vi "R4DOControl.vi"(8 "error constant":errorcluster, 11 "LabVIEW Web Service":refnum<class "Web Service.lvclass">) -> ()   [LabVIEW 2016]
uses:
  <vilib>/wsapi/Web Service.lvclass
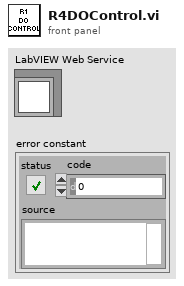
[diagram p1: front panel]
types:
  T1 = cluster{"Media Pump":bool, "Water Pump":bool, "Gas Pump":bool, "Effluent Pump":bool, "Release Pump":bool}
  T2 = cluster{"Set Point, mg/L":dbl, "Tolerance, mg/L":dbl, "N2 Valve Gain":dbl, "Air Valve Gain":dbl}
  T3 = cluster{"Signal, mA":dbl, "Value, UNITS HERE":dbl}
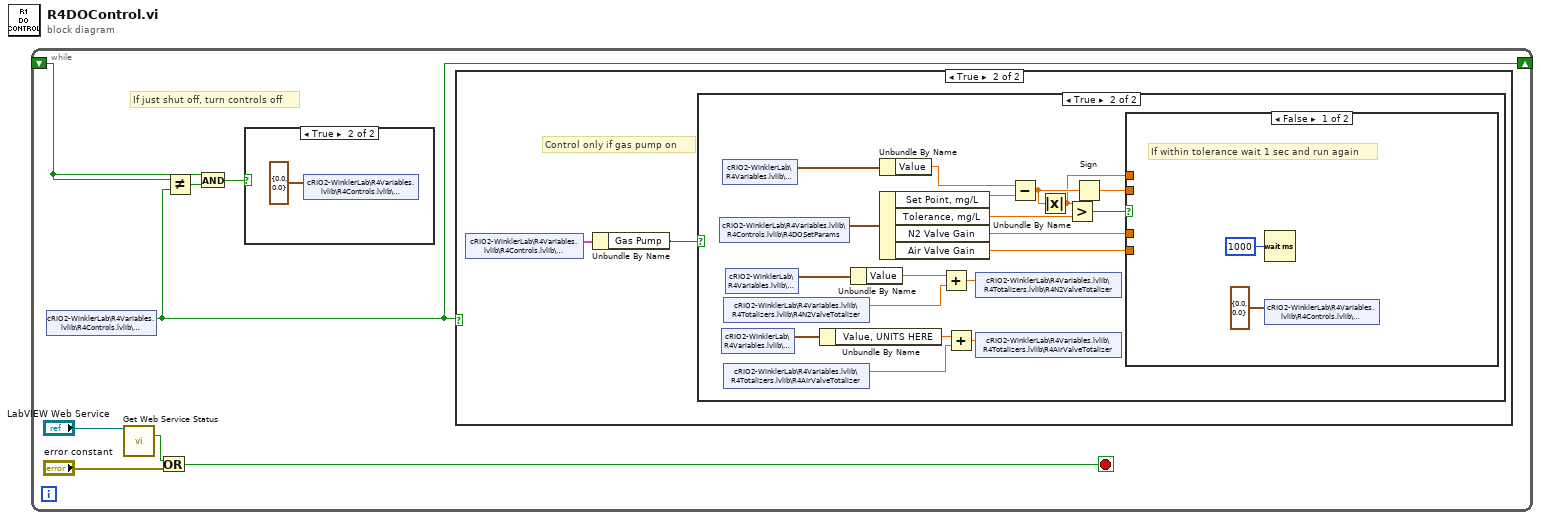
[diagram p0: block diagram]
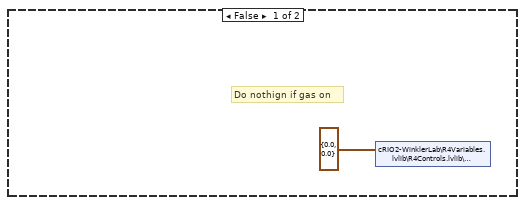
[diagram p4: hidden frame]
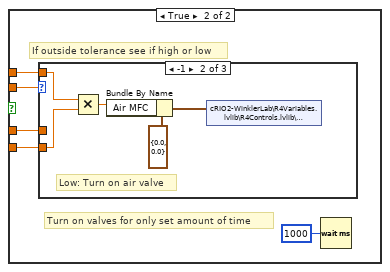
[diagram p5: hidden frame]
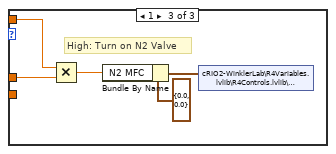
[diagram p7: hidden frame]
diagram:
  n1 = while {
    shift-right: [w1] -> _
    shift-left: _ -> [w2]
    stop <- w5 stop-if-true
    # "If just shut off, turn controls off"
    n2 = shared-variable "cRIO2-WinklerLab\\R4Variables.lvlib\\R4Controls.lvlib\\R4DOSwitch"() -> (w1:bool)  [unwired: 1 in, 1 out]
    n3 = call <vilib>:"Get Web Service Status.vi"("LabVIEW Web Service"="LabVIEW Web Service") -> ("service stopping?"=w8:bool)  [unwired: 12 in, 2 out]
    n4 = Or(x=w8, y="error constant") -> (x .or. y?=w5:bool)
    n5 = Not Equal?(x=w2, y=w1) -> (x != y?=w3:bool)
    n6 = And(x=w2, y=w3) -> (x .and. y?=w4:bool)
    n7 = case shown="True" w4 {
      frame False {
      }
      frame True {
        n8 = shared-variable "cRIO2-WinklerLab\\R4Variables.lvlib\\R4Controls.lvlib\\R4DOManual"(cluster{"Air MFC":dbl, "N2 MFC":dbl} {"Air MFC"=0.0, "N2 MFC"=0.0} ("R1DOManual")) -> ()  [unwired: 1 in, 1 out]
      }
    }
    n9 = case shown="True" w1 {
      frame False {
        # "Don't do anything if control is off"
      }
      frame True {
        # "Control only if gas pump on"
        n10 = shared-variable "cRIO2-WinklerLab\\R4Variables.lvlib\\R4Controls.lvlib\\R4SBRManual"() -> (w10:T1)  [unwired: 1 in, 1 out]
        n11 = Unbundle By Name(w10) -> ("Gas Pump"=w11:bool)
        n12 = case shown="True" w11 {
          frame False {
            # "Do nothign if gas on"
            n13 = shared-variable "cRIO2-WinklerLab\\R4Variables.lvlib\\R4Controls.lvlib\\R4DOManual"(cluster{"Air MFC":dbl, "N2 MFC":dbl} {"Air MFC"=0.0, "N2 MFC"=0.0} ("R1DOManual")) -> ()  [unwired: 1 in, 1 out]
          }
          frame True {
            n14 = shared-variable "cRIO2-WinklerLab\\R4Variables.lvlib\\R4Controls.lvlib\\R4DOSetParams"() -> (w20:T2)  [unwired: 1 in, 1 out]
            n15 = shared-variable "cRIO2-WinklerLab\\R4Variables.lvlib\\R4Signals.lvlib\\R4Air"() -> (w15:T3)  [unwired: 1 in, 1 out]
            n16 = shared-variable "cRIO2-WinklerLab\\R4Variables.lvlib\\R4Signals.lvlib\\R4DO"() -> (w18:cluster{"Signal":dbl, "Value":dbl})  [unwired: 1 in, 1 out]
            n17 = shared-variable "cRIO2-WinklerLab\\R4Variables.lvlib\\R4Totalizers.lvlib\\R4N2ValveTotalizer"() -> (w16:dbl)  [unwired: 1 in, 1 out]
            n18 = shared-variable "cRIO2-WinklerLab\\R4Variables.lvlib\\R4Totalizers.lvlib\\R4AirValveTotalizer"() -> (w19:dbl)  [unwired: 1 in, 1 out]
            n19 = shared-variable "cRIO2-WinklerLab\\R4Variables.lvlib\\R4Signals.lvlib\\R4N2"() -> (w17:cluster{"Signal":dbl, "Value":dbl})  [unwired: 1 in, 1 out]
            n20 = Unbundle By Name(w15) -> ("Value, UNITS HERE"=w22:dbl)
            n21 = Unbundle By Name(w17) -> ("Value"=w21:dbl)
            n22 = Unbundle By Name(w18) -> ("Value"=w31:dbl)
            n23 = Unbundle By Name(w20) -> ("Set Point, mg/L"=w30:dbl, "Tolerance, mg/L"=w29:dbl, "N2 Valve Gain"=w26:dbl, "Air Valve Gain"=w25:dbl)
            n24 = Add(x=w21, y=w16) -> (x+y=w14:dbl)
            n25 = Add(x=w22, y=w19) -> (x+y=w13:dbl)
            n26 = shared-variable "cRIO2-WinklerLab\\R4Variables.lvlib\\R4Totalizers.lvlib\\R4N2ValveTotalizer"(w14) -> ()  [unwired: 1 in, 1 out]
            n27 = shared-variable "cRIO2-WinklerLab\\R4Variables.lvlib\\R4Totalizers.lvlib\\R4AirValveTotalizer"(w13) -> ()  [unwired: 1 in, 1 out]
            n28 = Subtract(x=w31, y=w30) -> (x-y=w24:dbl)
            n29 = Absolute Value(x=w24) -> (abs(x)=w23:dbl)
            n30 = Greater?(x=w23, y=w29) -> (0:w28:bool)
            n31 = Sign(1:w24) -> (0:w27:dbl)
            n32 = case shown="False" w28 {
              tunnel: w27 -> [_ w38]
              tunnel: w26 -> [_ w37]
              tunnel: w25 -> [_ w36]
              tunnel: w23 -> [_ w35]
              frame False {
                # "If within tolerance wait 1 sec and run again"
                n33 = Wait (ms)(milliseconds to wait=u32 1000) -> ()  [unwired: 1 out]
                n34 = shared-variable "cRIO2-WinklerLab\\R4Variables.lvlib\\R4Controls.lvlib\\R4DOManual"(cluster{"Air MFC":dbl, "N2 MFC":dbl} {"Air MFC"=0.0, "N2 MFC"=0.0} ("R1DOManual")) -> ()  [unwired: 1 in, 1 out]
              }
              frame True {
                # "Turn on valves for only set amount of time"
                # "If outside tolerance see if high or low"
                n35 = case shown="-1" w38 {
                  tunnel: w36 -> [_ w40 _]
                  tunnel: w37 -> [_ _ w46]
                  tunnel: w35 -> [_ w41 w47]
                  frame 0, Default {
                    # "Unless tolerance is 0 this code\nshouldn't be accesible"
                  }
                  frame -1 {
                    # "Low: Turn on air valve"
                    n36 = Multiply(x=w41, y=w40) -> (x*y=w42:dbl)
                    n37 = Bundle By Name(cluster=cluster{"Air MFC":dbl, "N2 MFC":dbl} {"Air MFC"=0.0, "N2 MFC"=0.0} ("R1DOManual"), "Air MFC"=w42) -> (w39:cluster{"Air MFC":dbl, "N2 MFC":dbl})
                    n38 = shared-variable "cRIO2-WinklerLab\\R4Variables.lvlib\\R4Controls.lvlib\\R4DOManual"(w39) -> ()  [unwired: 1 in, 1 out]
                  }
                  frame 1 {
                    # "High: Turn on N2 Valve"
                    n39 = Multiply(x=w47, y=w46) -> (x*y=w45:dbl)
                    n40 = Bundle By Name(cluster=cluster{"Air MFC":dbl, "N2 MFC":dbl} {"Air MFC"=0.0, "N2 MFC"=0.0} ("R1DOManual"), "N2 MFC"=w45) -> (w44:cluster{"Air MFC":dbl, "N2 MFC":dbl})
                    n41 = shared-variable "cRIO2-WinklerLab\\R4Variables.lvlib\\R4Controls.lvlib\\R4DOManual"(w44) -> ()  [unwired: 1 in, 1 out]
                  }
                }
                n42 = Wait (ms)(milliseconds to wait=u32 1000) -> ()  [unwired: 1 out]
              }
            }
          }
        }
      }
    }
  }
